vi "q4 sum of digits.vi"() -> ()   [LabVIEW 2025]
panel:
  out "sum of digits":dbl
  in  "n":dbl
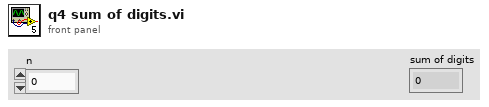
[diagram p1: front panel]
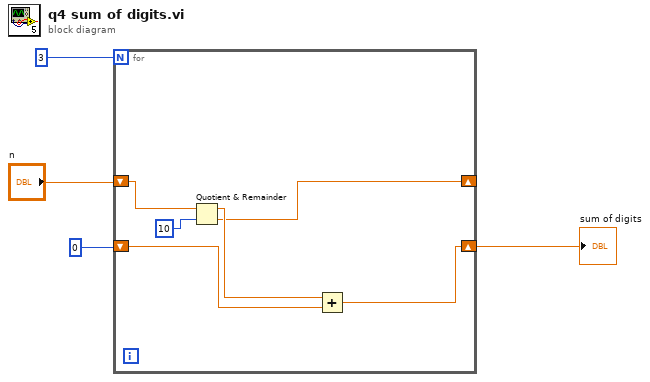
[diagram p0: block diagram]
diagram:
  n1 = for {
    N: 3 -> [_]
    shift-right: [w6] -> _
    shift-left: "n" -> [w10]
    shift-right: [w5] -> w1
    shift-left: 0 -> [w8]
    n2 = Quotient & Remainder(x=w10, y=10) -> (x-y*floor(x/y)=w7:dbl, floor(x/y)=w6:dbl)
    n3 = Add(x=w7, y=w8) -> (x+y=w5:dbl)
  }
  "sum of digits" <- w1
